vi "Starting Square Type.vi"(11 "MyTeam in":refnum<class "MyTeam.lvclass">) -> (2 "Square":refnum<class "Square.lvclass">, 3 "MyTeam out":refnum<class "MyTeam.lvclass">)   [LabVIEW 2020, in "SquareTeam.lvlib" / "MyTeam.lvclass"]
uses:
  MyTeam.lvclass
  SquareBattle/Square/Square.lvclass
  MySquare/MySquare.lvclass
  C:/dev/sol-squarebattle/SquareBattle/Square/Square.lvclass
  MyTeam.lvclass/MyTeam.ctl
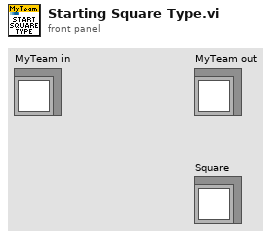
[diagram p1: front panel]
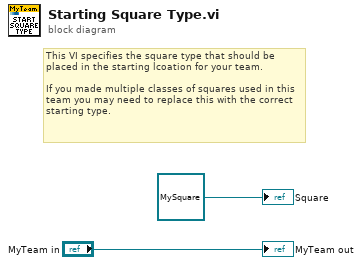
[diagram p0: block diagram]
diagram:
  # "This VI specifies the square type that should be placed in the starting lcoation for your team.\n\nIf you made multiple classes of squares used in this team you may need to replace this with the correct starting type."
  "MyTeam out" <- "MyTeam in"
  "Square" <- refnum<class "MySquare.lvclass"> refnum ("SquareTeam.lvlib:MySquare.lvclass")
